vi "zad1.vi"() -> (0 "Tablica 2d":dbl[][](array[numeric]))   [LabVIEW 2017]
panel:
  in  "liczba kolumn":dbl
  in  "liczba wierszy":dbl
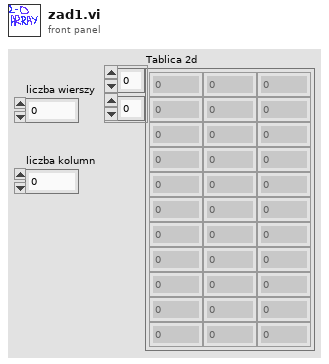
[diagram p1: front panel]
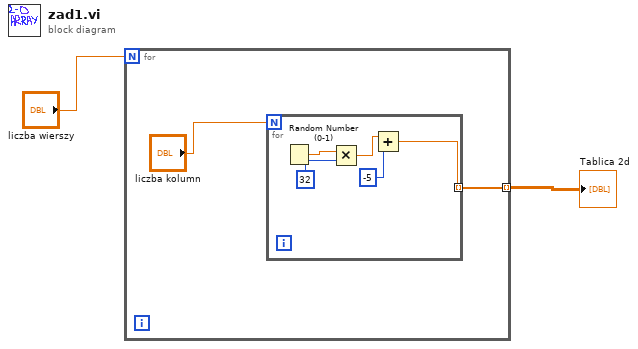
[diagram p0: block diagram]
diagram:
  n1 = for {
    N: "liczba wierszy" -> [_]
    tunnel: [w3] -> w1 mode=indexing
    n2 = for {
      N: "liczba kolumn" -> [_]
      tunnel: [w5] -> w3 mode=indexing
      n3 = Random Number (0-1)() -> (number: 0 to 1=w9:dbl)
      n4 = Multiply(x=w9, y=32) -> (x*y=w7:dbl)
      n5 = Add(x=w7, y=-5) -> (x+y=w5:dbl)
    }
  }
  "Tablica 2d" <- w1
